vi "PathPlanner_ReplanningConfig_New.vi"(8 "dynamicReplanningErrorSpikeThreshold":dbl=0.25, 9 "dynamicReplanningTotalErrorThreshold":dbl=1.0, 10 "enableDynamicReplanning":bool, 11 "enableInitialReplanning":bool=TRUE) -> (3 "ReplanningConfig":T1)   [LabVIEW 2019, in "PathPlanner24.lvlib"]
doc: "Create a path replanning configuration\n\nInputs:\n - EnableInitialReplanning - boolean Should the path be replanned at the start of path following if the robot is not already at the starting point? (Optional. Default: TRUE)\n - EnableDynamicReplanning boolean - Should the path be replanned if the error grows too large or if a large error spike happens while following the path? (Optional. Default: FALSE)\n - DynamicReplanningTotalErrorThreshold - double - The total error threshold, in meters, that will cause the path to be replanned (Optional. Default: 1.0)\n - DynamicReplanningErrorSpikeThreshold - double - The error spike threshold, in meters, that will cause the path to be replanned. (Optional. Default: 0.25)\n\nOutputs:\n - ReplanningConfig - cluster - created data cluster"
uses:
  PathPlanner24.lvlib
  TypeDef/PathPlannerReplanningConfig.ctl
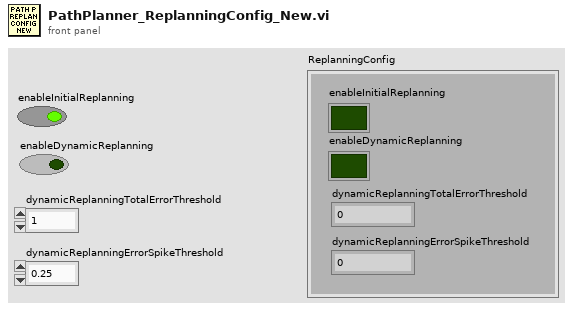
[diagram p1: front panel]
types:
  T1 = typedef "PathPlanner24.lvlib/PathPlannerReplanningConfig.ctl" = cluster{"enableInitialReplanning":bool, "enableDynamicReplanning":bool, "dynamicReplanningTotalErrorThreshold":dbl, "dynamicReplanningErrorSpikeThreshold":dbl}
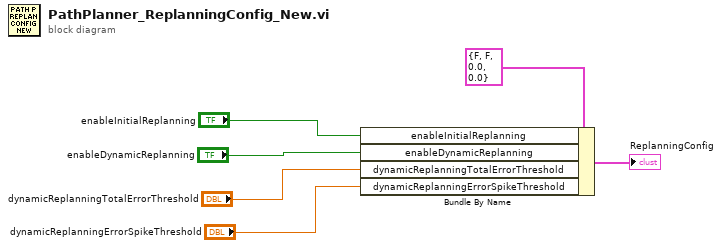
[diagram p0: block diagram]
diagram:
  n1 = Bundle By Name(cluster=T1 {"enableInitialReplanning"=FALSE, "enableDynamicReplanning"=FALSE, "dynamicReplanningTotalErrorThreshold"=0.0, "dynamicReplanningErrorSpikeThreshold"=0.0} ("ReplanningConfig"), "enableInitialReplanning"="enableInitialReplanning", "enableDynamicReplanning"="enableDynamicReplanning", "dynamicReplanningTotalErrorThreshold"="dynamicReplanningTotalErrorThreshold", "dynamicReplanningErrorSpikeThreshold"="dynamicReplanningErrorSpikeThreshold") -> (→"ReplanningConfig":T1)
